vi "Handle Message.vi"(5 "Stack ID":u8, 7 "Function ID":u8, 8 "error in (no error)":errorcluster, 10 "Data":string, 11 "Dual Relay Bricklet in":refnum<class "Dual Relay Bricklet.lvclass">) -> (0 "error out":errorcluster, 1 "Send Answer":bool, 2 "Answer":variant, 3 "Dual Relay Bricklet out":refnum<class "Dual Relay Bricklet.lvclass">)   [LabVIEW 2011, in "Tinkerforge.lvlib" / "Dual Relay Bricklet.lvclass"]
doc: "This VI is the child implementation of \"Handle Message.vi\" and processes all responses for this device type."
uses:
  Dual Relay Bricklet.lvclass
  Type Definitions/Relay States.ctl
  Device/Device.lvclass
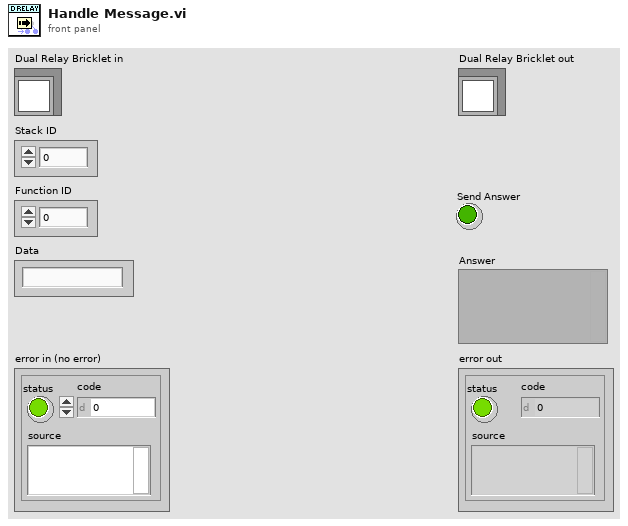
[diagram p1: front panel]
types:
  T1 = typedef "Tinkerforge.lvlib/Dual Relay Bricklet.lvclass/Relay States.ctl" = cluster{"relay 1":bool, "relay 2":bool}
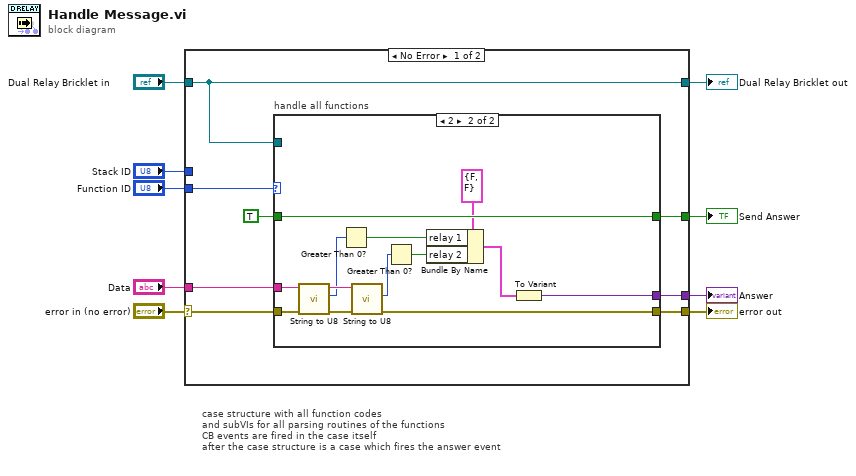
[diagram p0: block diagram]
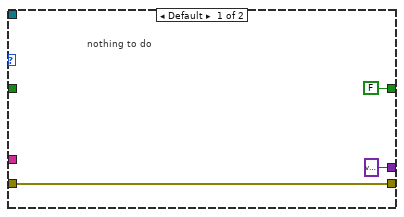
[diagram p2: hidden frame]
diagram:
  # "case structure with all function codes\nand subVIs for all parsing routines of the functions\nCB events are fired in the case itself\nafter the case structure is a case which fires the answer event"
  n1 = case shown="No Error" "error in (no error)" {
    selector: "error in (no error)" -> [w14 w34]
    tunnel: "Dual Relay Bricklet in" -> [w17 w35]
    tunnel: "Stack ID" -> [_ _]
    tunnel: "Function ID" -> [w16 _]
    tunnel: "Data" -> [w13 _]
    tunnel: [w17 w35] -> w4
    tunnel: [w12 w34] -> w3
    tunnel: [w11 _] -> w2
    tunnel: [w10 _] -> w1
    frame No Error {
      n2 = case "handle all functions" shown="2" w16 {
        tunnel: w14 -> [w20 w32]
        tunnel: TRUE -> [_ w33]
        tunnel: [FALSE w33] -> w10
        tunnel: [w20 w21] -> w12
        tunnel: [variant ("Variant") w22] -> w11
        tunnel: w17 -> [_ _]
        tunnel: w13 -> [_ w31]
        frame Default {
          # "nothing to do"
        }
        frame 2 {
          n3 = call "String to U8.vi"("Error In"=w32, "String"=w31) -> ("Error Out"=w30:errorcluster, "U8"=w28:u8, "rest of String"=w29:string)  [unwired: 7 in]
          n4 = Greater Than 0?(x=w28) -> (x > 0?=w25:bool)
          n5 = call "String to U8.vi"("Error In"=w30, "String"=w29) -> ("Error Out"=w21:errorcluster, "U8"=w27:u8)  [unwired: 7 in, 1 out]
          n6 = Greater Than 0?(x=w27) -> (x > 0?=w24:bool)
          n7 = Bundle By Name(cluster=T1 {"relay 1"=FALSE, "relay 2"=FALSE} ("Relay States"), "relay 1"=w25, "relay 2"=w24) -> (w23:T1)
          n8 = To Variant(anything=w23) -> (Variant=w22:variant)
        }
      }
    }
    frame Error {
    }
  }
  "error out" <- w3
  "Dual Relay Bricklet out" <- w4
  "Answer" <- w2
  "Send Answer" <- w1
